vi "basic_settings.vi"(0 "VISA resource name":refnum<visa-resource-name>="TRIG", 1 "Burst enable?":bool, 2 "burst period (s)":dbl, 3 "burst count":i32, 5 "power level":string, 7 "polarity":bool[](array[boolean]), 11 "error in (no error)":errorcluster) -> (4 "VISA resource name out":refnum<visa-resource-name>, 15 "error out":errorcluster)   [LabVIEW 2011]
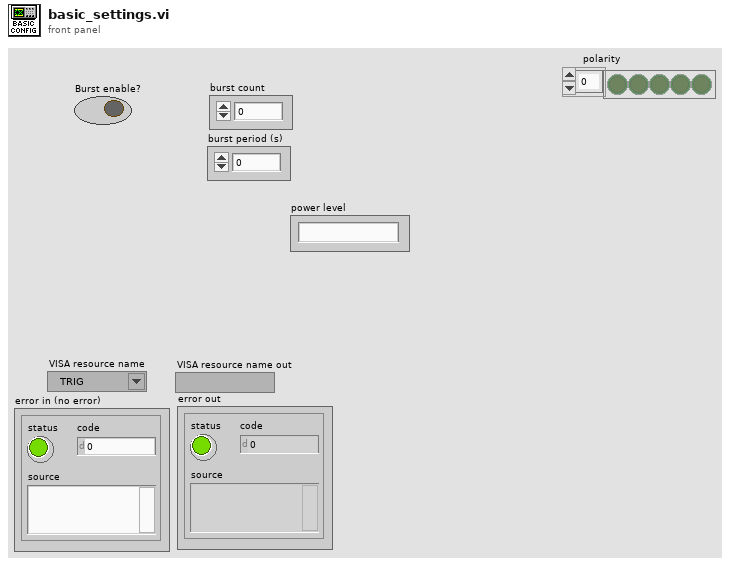
[diagram p1: front panel]
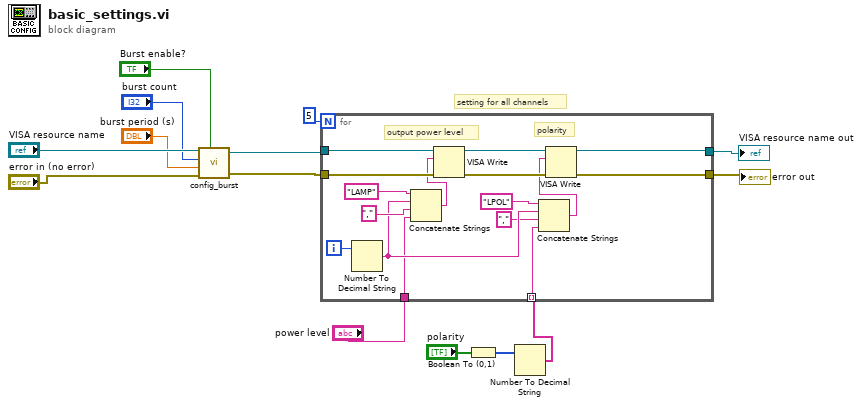
[diagram p0: block diagram]
diagram:
  # "setting for all channels"
  n1 = call "config_burst.vi"("VISA resource name"="VISA resource name", "burst count"="burst count", "burst period (s)"="burst period (s)", "error in (no error)"="error in (no error)", "Burst enable?"="Burst enable?") -> ("VISA resource name out"=w7:refnum<visa-resource-name>, "error out"=w8:errorcluster)  [unwired: 1 in]
  n2 = Boolean To (0,1)(Boolean="polarity") -> (0, 1=w3:i16[])
  n3 = Number To Decimal String(number=w3) -> (decimal integer string=w1:string[])  [unwired: 1 in]
  n4 = for {
    N: 5 -> [_]
    tunnel: w7 -> [w29]
    tunnel: [w22] -> w14
    tunnel: w8 -> [w28]
    tunnel: [w23] -> w13
    tunnel: w1 -> [w18] mode=indexing
    tunnel: "power level" -> [w16]
    i -> [w15]
    # "polarity"
    # "output power level"
    n5 = Number To Decimal String(number=w15) -> (decimal integer string=w20:string)  [unwired: 1 in]
    n6 = Concatenate Strings("LAMP" ("Query 2"), w20, "," ("Query 2"), w16) -> (w25:string)
    n7 = VISA Write(VISA resource name=w29, write buffer=w25, error in (no error)=w28) -> (VISA resource name out=w24:refnum<visa-resource-name>, error out=w27:errorcluster)  [unwired: 1 out]
    n8 = Concatenate Strings("LPOL" ("Query 2"), w20, "," ("string"), w18) -> (w19:string)
    n9 = VISA Write(VISA resource name=w24, write buffer=w19, error in (no error)=w27) -> (VISA resource name out=w22:refnum<visa-resource-name>, error out=w23:errorcluster)  [unwired: 1 out]
  }
  "VISA resource name out" <- w14
  "error out" <- w13
